vi "Perform Diagnostic Loop Back Test.vi"(8 "error in (no error)":errorcluster, 10 "Loop Back Test Type (0: Digital Bus)":i32(ring) items=["Digital Bus", "Digital Bus Loop Back Fixture", "N5102A", "Single Ended IO Dual 40 Pin Device"], 11 "VISA resource name":refnum<visa-resource-name>) -> (0 "error out":errorcluster, 2 "Test Result":string, 3 "VISA resource name out":refnum<visa-resource-name>)   [LabVIEW 2018, in "Agilent PSG MXG Series.lvlib"]
doc: "Selects and executes a loop back test that validates the integrity of digital data and returns a pass or fail condition.\n\n<b>Notes:</b>\n(1) This VI is valid only in N5172B/82B that installs with <B>Option 003</B> or <B>Option 004</B> or <B>both</B>. \n(2) A N5102A must be attached to the rear panel LVDS port to execute this VI successfully."
uses:
  Agilent PSG MXG Series.lvlib
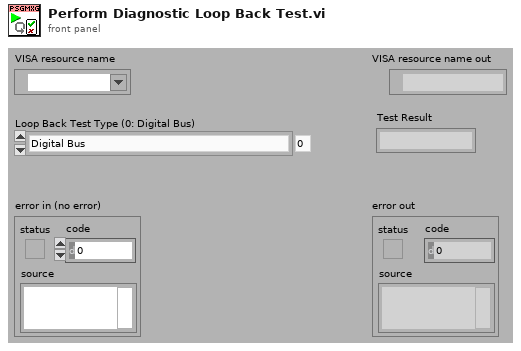
[diagram p1: front panel]
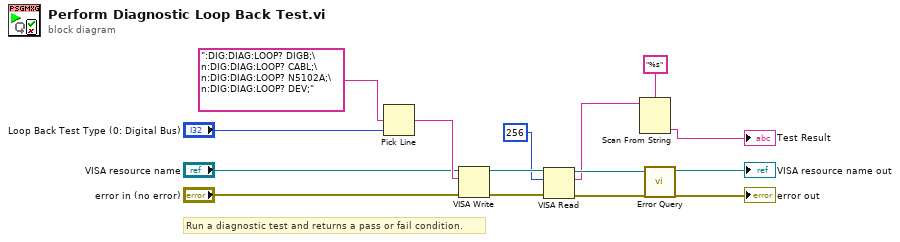
[diagram p0: block diagram]
diagram:
  # "Run a diagnostic test and returns a pass or fail condition."
  n1 = Pick Line(multi-line string=":DIG:DIAG:LOOP? DIGB;\n:DIG:DIAG:LOOP? CABL;\n:DIG:DIAG:LOOP? N5102A;\n:DIG:DIAG:LOOP? DEV;", line index="Loop Back Test Type (0: Digital Bus)") -> (output string=w13:string)  [unwired: 1 in]
  n2 = VISA Write(VISA resource name="VISA resource name", write buffer=w13, error in (no error)="error in (no error)") -> (VISA resource name out=w8:refnum<visa-resource-name>, error out=w7:errorcluster)  [unwired: 1 out]
  n3 = VISA Read(VISA resource name=w8, byte count=u32 256, error in (no error)=w7) -> (VISA resource name out=w6:refnum<visa-resource-name>, read buffer=w3:string, error out=w5:errorcluster)  [unwired: 1 out]
  n4 = Scan From String(format string="%s", input string=w3) -> (output 1=→"Test Result":string)  [unwired: 3 in, 3 out]
  n5 = call "Error Query.vi"("error in (no error)"=w5, "VISA resource name"=w6) -> ("error out"=→"error out":errorcluster, "VISA resource name out"=→"VISA resource name out":refnum<visa-resource-name>)  [unwired: 6 in, 2 out]
